vi "Measure Output.vi"(8 "error in":errorcluster, 11 "69X_79X in":refnum<class "79XRP.lvclass">) -> (0 "error out":errorcluster, 1 "Current":dbl[](array[numeric]), 2 "Voltage":dbl[](array[numeric]), 3 "69X_79X out":refnum<class "79XRP.lvclass">)   [LabVIEW 2019, in "79XRP.lvlib" / "79XRP.lvclass"]
uses:
  Library/79XRP.lvclass
  Library/79XRP.lvclass/79XRP.ctl
  <instrlib>/Keysight RP7900 Series/Keysight RP7900 Series.lvlib
  builds/Engine/Engine.lvlibp/Project/Engine.lvclass
  C:/Users/Public/Documents/Development/builds/Engine/Engine.lvlibp/Project/Engine.lvclass
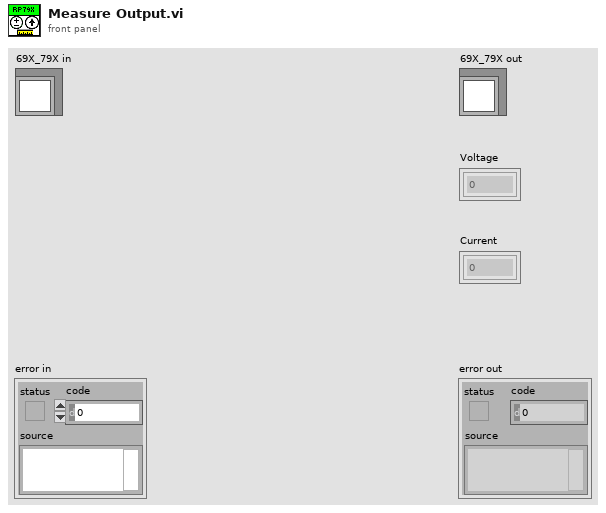
[diagram p1: front panel]
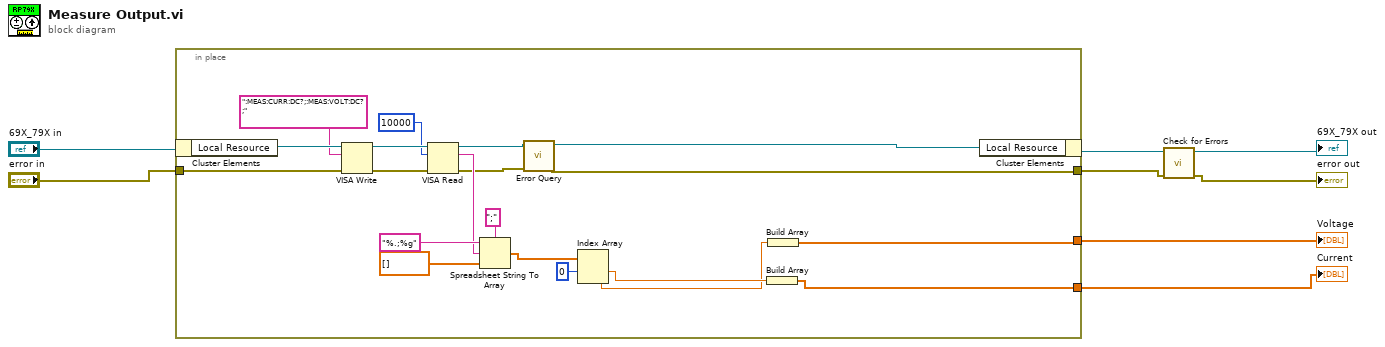
[diagram p0: block diagram]
diagram:
  n1 = in-place {
    in-place-border: "error in" -> [w19]
    in-place-border: [w9] -> w2
    in-place-border: [w11] -> w6
    in-place-border: [w13] -> w5
    n2 = in-place-cluster #1("69X_79X in") -> ("Local Resource"=w28:refnum<visa-resource-name>)
    n3 = VISA Write(VISA resource name=w28, write buffer=":MEAS:CURR:DC?;:MEAS:VOLT:DC?;", error in (no error)=w19) -> (VISA resource name out=w25:refnum<visa-resource-name>, error out=w26:errorcluster)  [unwired: 1 out]
    n4 = VISA Read(VISA resource name=w25, byte count=u32 10000, error in (no error)=w26) -> (VISA resource name out=w18:refnum<visa-resource-name>, read buffer=w21:string, error out=w17:errorcluster)  [unwired: 1 out]
    n5 = Spreadsheet String To Array(delimiter (Tab)=";", format string="%.;%g", spreadsheet string=w21, array type (2D Dbl)=dbl[] []) -> (array=w16:dbl[])
    n6 = call <instrlib>:"Error Query.vi"("error in (no error)"=w17, "VISA resource name"=w18) -> ("error out"=w9:errorcluster, "VISA resource name out"=w10:refnum<visa-resource-name>)  [unwired: 6 in, 2 out]
    n7 = Index Array(array=w16, index #1=0 ("index")) -> (element #1=w14:dbl, element #2=w12:dbl)  [unwired: 1 in]
    n8 = Build Array(w14) -> (w13:dbl[])
    n9 = Build Array(w12) -> (w11:dbl[])
    n10 = in-place-cluster #1("Local Resource"=w10) -> (w4:refnum<class "79XRP.lvclass">)
  }
  "Current" <- w5
  "Voltage" <- w6
  n11 = call "Check for Errors.vi"("error in"=w2, "Engine in"=w4) -> ("error out"=→"error out":errorcluster, "Engine out"=→"69X_79X out":refnum<class "79XRP.lvclass">)  [unwired: 8 in]
